vi "List Procs.vi"(4 "error in (no error)":errorcluster) -> (0 "error out":errorcluster, 1 "ProcId's":i32[](array[numeric]), 2 "FullModuleNames":string[](array[string]), 3 "ProcessNames":string[](array[string]))   [LabVIEW 2011]
uses:
  KERNEL32.DLL
  psapi.dll
panel:
  out "Procs":i32
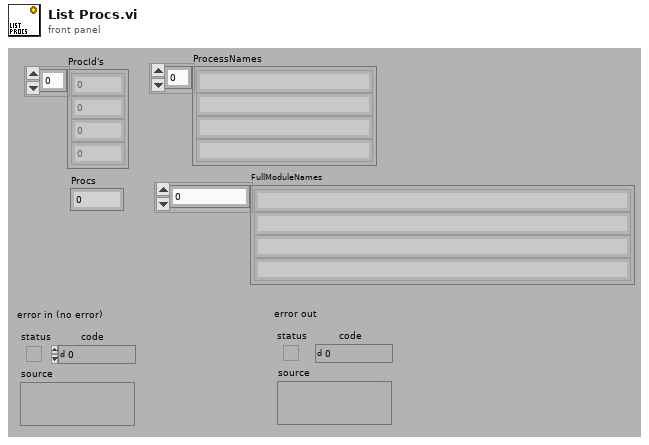
[diagram p1: front panel]
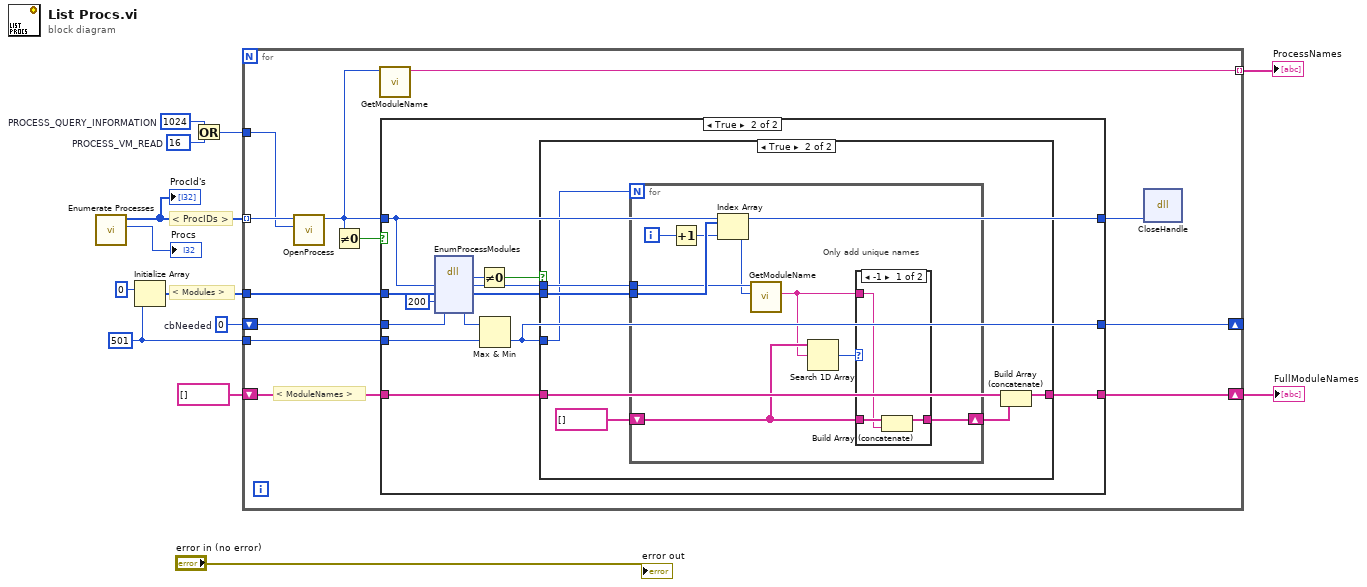
[diagram p0: block diagram]
diagram:
  w3 = 16  # PROCESS_VM_READ
  w4 = 1024  # PROCESS_QUERY_INFORMATION
  w12 = 0  # cbNeeded
  w11 = 501 ("dimension size")
  # "< Modules >"
  # "< ProcIDs >"
  n1 = call "Enumerate Processes.vi"() -> ("Process Count"=→"Procs":i32, "Process IDs"=w7:i32[])  [unwired: 1 in, 5 out]
  "ProcId's" <- w7
  n2 = Initialize Array(0 ("cbNeeded"), w11) -> (w9:i32[])
  n3 = Or(x=w4, y=w3) -> (x .or. y?=w2:i32)
  n4 = for {
    tunnel: w7 -> [w16] mode=indexing
    shift-right: [w22] -> _
    shift-left: w12 -> [w24]
    tunnel: w11 -> [w23]
    shift-right: [w20] -> w8
    shift-left: string[] [] -> [w21]
    tunnel: w9 -> [w19]
    tunnel: [w17] -> w5 mode=indexing
    tunnel: w2 -> [w14]
    # "< ModuleNames >"
    n5 = call "OpenProcess.vi"("dwDesiredAccesses (0)"=w14, "dwProcessId (0)"=w16) -> ("hProcess"=w15:i32)  [unwired: 2 in, 3 out]
    n6 = Not Equal To 0?(x=w15) -> (x != 0?=w25:bool)
    n7 = call "GetModuleName.vi"("hProcess (0)"=w15) -> ("Module Name"=w17:string)  [unwired: 2 in, 4 out]
    n8 = case shown="True" w25 {
      tunnel: w19 -> [_ w40]
      tunnel: w24 -> [w28 w39]
      tunnel: w23 -> [_ w37]
      tunnel: w15 -> [w26 w29]
      tunnel: [w28 w30] -> w22
      tunnel: w21 -> [w27 w32]
      tunnel: [w27 w31] -> w20
      tunnel: [w26 w29] -> w18
      frame False {
      }
      frame True {
        n9 = dll-call lib="psapi.dll" fn="EnumProcessModules"("hProcess"=w29, "lphModule"=w40, "cb"=200, "cbNeeded"=w39) -> (w36:i32, "hProcess"=w34:i32, "lphModule"=w33:i32[], "cbNeeded"=w38:i32)  [unwired: 4 in, 2 out]
        n10 = Not Equal To 0?(x=w36) -> (x != 0?=w35:bool)
        n11 = Max & Min(x=w38, y=w37) -> (min(x,y)=w30:i32)  [unwired: 1 out]
        n12 = case shown="True" w35 {
          tunnel: w34 -> [_ w49]
          tunnel: w33 -> [_ w46]
          tunnel: w32 -> [w42 w48]
          tunnel: [w42 w47] -> w31
          tunnel: w30 -> [_ w43]
          frame False {
          }
          frame True {
            n13 = for {
              N: w43 -> [_]
              tunnel: w49 -> [w52]
              tunnel: w46 -> [w58]
              shift-right: [w53] -> w44
              shift-left: string[] [] -> [w54]
              i -> [w57]
              # "Only add unique names"
              n14 = Increment(x=w57) -> (x+1=w56:i32)
              n15 = Index Array(array=w58, index=w56) -> (element=w51:i32)
              n16 = call "GetModuleName.vi"("hModule (0)"=w51, "hProcess (0)"=w52) -> ("Full Module Name"=w50:string)  [unwired: 1 in, 4 out]
              n17 = Search 1D Array(1D array=w54, element=w50) -> (index of element=w55:i32)  [unwired: 1 out]
              n18 = case shown="-1" w55 {
                tunnel: w54 -> [w61 w62]
                tunnel: [w59 w62] -> w53
                tunnel: w50 -> [w60 _]
                frame -1 {
                  n19 = Build Array (concatenate)(w61, w60) -> (w59:string[])
                }
                frame 0.., Default {
                }
              }
            }
            n20 = Build Array (concatenate)(w48, w44) -> (w47:string[])
          }
        }
      }
    }
    n21 = dll-call lib="KERNEL32.DLL" fn="CloseHandle"("Handle"=w18) -> ()  [unwired: 4 in, 3 out]
  }
  "FullModuleNames" <- w8
  "ProcessNames" <- w5
  "error out" <- "error in (no error)"
